vi "Loop Async.vi"(10 "ExecAnchor":refnum<class "ExecAnchor.lvclass">, 11 "HistorianCharting in":refnum<class "HistorianCharting.lvclass">) -> ()   [LabVIEW 2020, in "VolatusGUIElements.lvlib" / "HistorianCharting.lvclass"]
uses:
  HistorianCharting.lvclass
  lv-exec-anchor/ExecAnchor/ExecAnchor.lvclass
  HistorianCharting.lvclass/HistorianCharting.ctl
  <vilib>/dlg_ctls.llb/Space Constant.vi
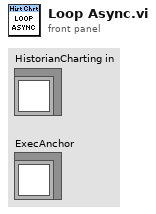
[diagram p1: front panel]
types:
  T1 = cluster{"Event Reg":refnum<event-registration>, "Event Reg":refnum<event-registration>, "Group Events":refnum<event-registration>}
  T2 = typedef "VolatusGUIElements.lvlib/HistorianCharting.lvclass/Buffer Info.ctl" = cluster{"Buffer":refnum<class "Group Buffer DBL.lvclass">, "Channels":string[], "Plot Indices":i32[]}
  T3 = typedef "VolatusGUI.lvlib/Historian Charting Manager.lvclass/Plot Group Config.ctl" = cluster{"Name":string, "X-Axis Type":T4, "X-Axis Channel":string, "Plots":T5[], "Lock Now":bool, "Time":string, "Swap Axes":bool}
  T4 = typedef "VolatusGUI.lvlib/Historian Charting Manager.lvclass/X-Axis Type.ctl" = enum16{"Time", "Channel"}
  T5 = typedef "VolatusGUI.lvlib/Historian Charting Manager.lvclass/Plot Config.ctl" = cluster{"Channel":string, "Visible":bool, "Color":u32, "Scale":T6}
  T6 = typedef "VolatusGUI.lvlib/Historian Charting Manager.lvclass/Scale.ctl" = enum16{"Left", "Right"}
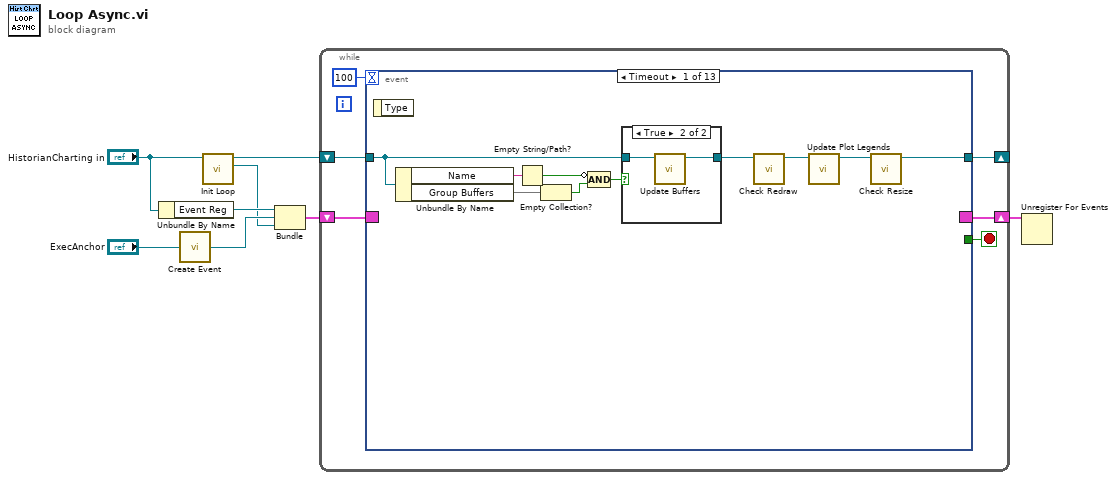
[diagram p0: block diagram]
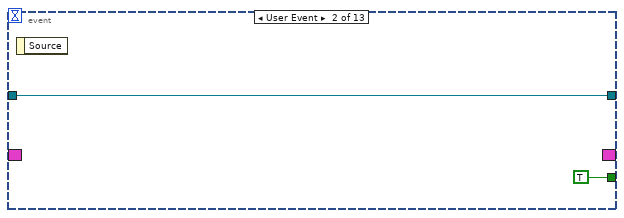
[diagram p3: hidden frame]
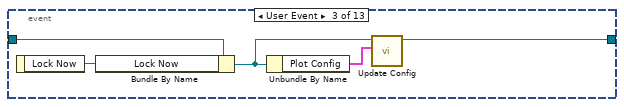
[diagram p4: hidden frame]
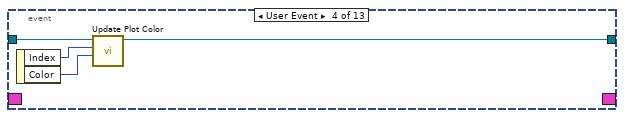
[diagram p5: hidden frame]
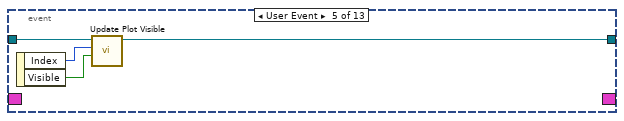
[diagram p6: hidden frame]
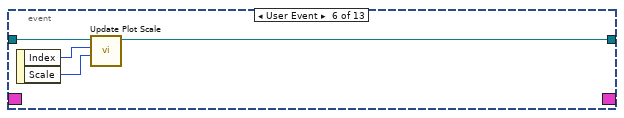
[diagram p7: hidden frame]
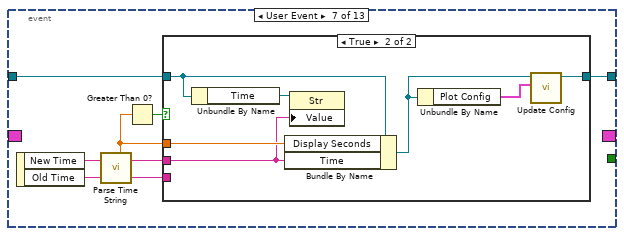
[diagram p8: hidden frame]
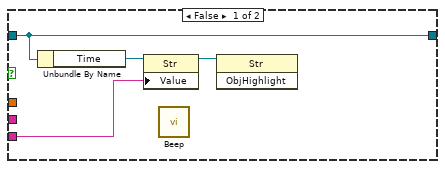
[diagram p9: hidden frame]
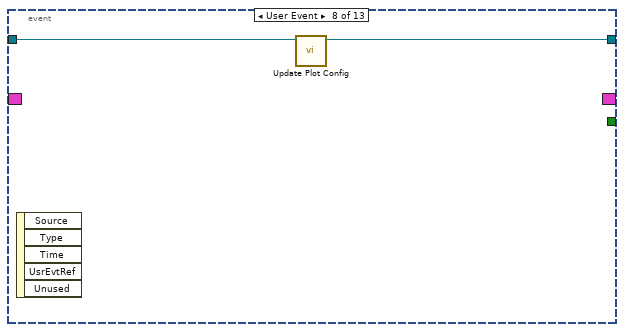
[diagram p10: hidden frame]
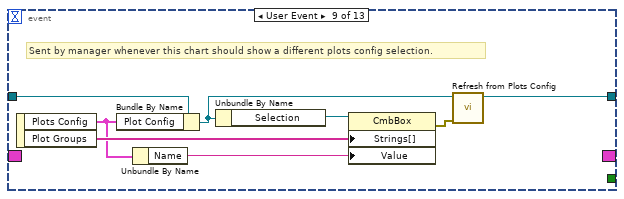
[diagram p11: hidden frame]
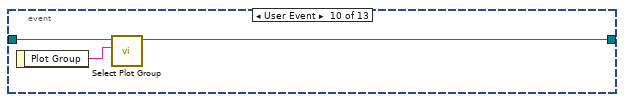
[diagram p12: hidden frame]
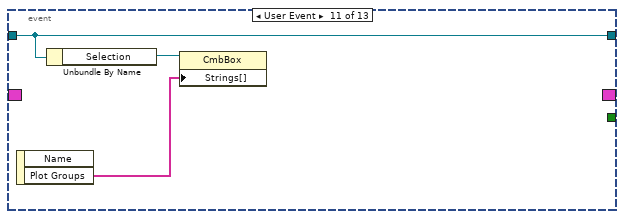
[diagram p13: hidden frame]
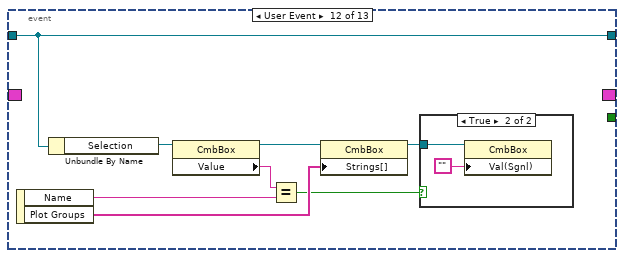
[diagram p14: hidden frame]
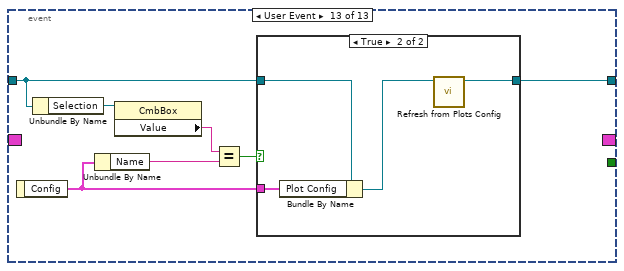
[diagram p16: hidden frame]
diagram:
  n1 = Unbundle By Name("HistorianCharting in") -> ("Event Reg"=w6:refnum<event-registration>)
  n2 = call "Create Event.vi"("ExecAnchor in"="ExecAnchor") -> ("Event Reg"=w5:refnum<event-registration>)  [unwired: 3 in, 1 out]
  n3 = call "Init Loop.vi"("HistorianCharting in"="HistorianCharting in") -> ("Group Events"=w1:refnum<event-registration>, "HistorianCharting out"=w2:refnum<class "HistorianCharting.lvclass">)  [unwired: 8 in, 1 out]
  n4 = Bundle("Event Reg"=w6, "Event Reg"=w5, "Group Events"=w1) -> (w4:T1)  [unwired: 1 in]
  n5 = while {
    shift-right: [w12] -> _
    shift-left: w2 -> [w13]
    shift-right: [w10] -> w3
    shift-left: w4 -> [w11]
    stop <- w9 stop-if-true
    n6 = event shown="[0] Timeout" {
      selector: w11 -> [_ _ _ _ _ _ _ _ _ _ _ _ _]
      dyn-events: [_ _ _ _ _ _ _ _ _ _ _ _ _] -> w10
      timeout: 100 -> [_ _ _ _ _ _ _ _ _ _ _ _ _]
      tunnel: w13 -> [w18 w29 w34 w38 w42 w46 w49 w66 w74 w77 w80 w87 w94]
      tunnel: [w15 w29 w31 w37 w41 w45 w48 w65 w73 w75 w80 w87 w91] -> w12
      tunnel: [_ TRUE _ _ _ _ _ _ _ _ _ _ _] -> w9
      event Timeout {
        n7 = event-data() -> ()  [unwired: 1 in, 1 out]
        n8 = Unbundle By Name(w18) -> ("Name"=w22:string, "Group Buffers"=w21:map{string, T2})
        n9 = Empty String/Path?(string/path=w22) -> (empty?=w20:bool)
        n10 = Empty Collection?(1:w21) -> (0:w19:bool)
        n11 = Compound Arithmetic op=AND(invert w20, w19) -> (w17:bool)
        n12 = case shown="True" w17 {
          tunnel: w18 -> [w25 w27]
          tunnel: [w25 w26] -> w16
          frame False {
          }
          frame True {
            n13 = call "Update Buffers.vi"("HistorianCharting in"=w27) -> ("HistorianCharting out"=w26:refnum<class "HistorianCharting.lvclass">)  [unwired: 9 in, 1 out]
          }
        }
        n14 = call "Check Redraw.vi"("HistorianCharting in"=w16) -> ("HistorianCharting out"=w24:refnum<class "HistorianCharting.lvclass">)  [unwired: 9 in, 1 out]
        n15 = call "Update Plot Legends.vi"("HistorianCharting in"=w24) -> ("HistorianCharting out"=w23:refnum<class "HistorianCharting.lvclass">)  [unwired: 9 in, 1 out]
        n16 = call "Check Resize.vi"("HistorianCharting in"=w23) -> ("HistorianCharting out"=w15:refnum<class "HistorianCharting.lvclass">)  [unwired: 9 in, 1 out]
      }
      event User Event {
        n17 = event-data() -> ()  [unwired: 1 in, 1 out]
      }
      event User Event {
        n18 = event-data() -> ("Lock Now"=w33:bool)  [unwired: 1 in]
        n19 = Bundle By Name(cluster=w34, "Lock Now"=w33) -> (w32:refnum<class "HistorianCharting.lvclass">)
        n20 = Unbundle By Name(w32) -> ("Plot Config"=w30:T3)
        n21 = call "Update Config.vi"("Config"=w30, "HistorianCharting in"=w32) -> ("HistorianCharting out"=w31:refnum<class "HistorianCharting.lvclass">)  [unwired: 8 in, 1 out]
      }
      event User Event {
        n22 = event-data() -> ("Index"=w36:i32, "Color"=w35:u32)  [unwired: 1 in]
        n23 = call "Update Plot Color.vi"("Color"=w35, "Index"=w36, "HistorianCharting in"=w38) -> ("HistorianCharting out"=w37:refnum<class "HistorianCharting.lvclass">)  [unwired: 7 in, 1 out]
      }
      event User Event {
        n24 = event-data() -> ("Index"=w40:i32, "Visible"=w39:bool)  [unwired: 1 in]
        n25 = call "Update Plot Visible.vi"("Visible"=w39, "Index"=w40, "HistorianCharting in"=w42) -> ("HistorianCharting out"=w41:refnum<class "HistorianCharting.lvclass">)  [unwired: 7 in, 1 out]
      }
      event User Event {
        n26 = event-data() -> ("Index"=w44:i32, "Scale"=w43:T6)  [unwired: 1 in]
        n27 = call "Update Plot Scale.vi"("Scale"=w43, "Index"=w44, "HistorianCharting in"=w46) -> ("HistorianCharting out"=w45:refnum<class "HistorianCharting.lvclass">)  [unwired: 7 in, 1 out]
      }
      event User Event {
        n28 = event-data() -> ("New Time"=w53:string, "Old Time"=w47:string)  [unwired: 1 in]
        n29 = call "Parse Time String.vi"("Time String"=w53) -> ("Seconds"=w51:dbl, "Normalized String"=w52:string)  [unwired: 5 in]
        n30 = Greater Than 0?(x=w51) -> (x > 0?=w50:bool)
        n31 = case shown="True" w50 {
          tunnel: w52 -> [_ w61]
          tunnel: w51 -> [_ w64]
          tunnel: w49 -> [w57 w62]
          tunnel: [w57 w60] -> w48
          tunnel: w47 -> [w54 _]
          frame False {
            n32 = Unbundle By Name(w57) -> ("Time"=w56:refnum<vi>)
            n33 = property class="Str"(reference=w56, "Value"=w54) -> (reference out=w55:refnum<vi>)  [unwired: 1 in, 1 out]
            n34 = call <vilib>:"Beep.vi"() -> ()  [unwired: 12 in]
            n35 = invoke class="Str" method="ObjHighlight"(reference=w55) -> ()  [unwired: 2 in, 3 out]
          }
          frame True {
            n36 = Unbundle By Name(w62) -> ("Time"=w63:refnum<vi>)
            n37 = Bundle By Name(cluster=w62, "Display Seconds"=w64, "Time"=w61) -> (w59:refnum<class "HistorianCharting.lvclass">)
            n38 = property class="Str"(reference=w63, "Value"=w61) -> ()  [unwired: 1 in, 2 out]
            n39 = Unbundle By Name(w59) -> ("Plot Config"=w58:T3)
            n40 = call "Update Config.vi"("Config"=w58, "HistorianCharting in"=w59) -> ("HistorianCharting out"=w60:refnum<class "HistorianCharting.lvclass">)  [unwired: 8 in, 1 out]
          }
        }
      }
      event User Event {
        n41 = event-data() -> ()  [unwired: 1 in, 5 out]
        n42 = call "Update Plot Config.vi"("HistorianCharting in"=w66) -> ("HistorianCharting out"=w65:refnum<class "HistorianCharting.lvclass">)  [unwired: 9 in, 1 out]
      }
      event User Event {
        # "Sent by manager whenever this chart should show a different plots config selection."
        n43 = event-data() -> ("Plots Config"=w68:T3, "Plot Groups"=w69:string[])  [unwired: 1 in]
        n44 = Bundle By Name(cluster=w74, "Plot Config"=w68) -> (w70:refnum<class "HistorianCharting.lvclass">)
        n45 = Unbundle By Name(w68) -> ("Name"=w67:string)
        n46 = Unbundle By Name(w70) -> ("Selection"=w72:refnum<vi>)
        n47 = property class="CmbBox"(reference=w72, "Strings[]"=w69, "Value"=w67) -> (error out=w71:errorcluster)  [unwired: 1 in, 1 out]
        n48 = call "Refresh from Plots Config.vi"("error in (no error)"=w71, "HistorianCharting in"=w70) -> ("HistorianCharting out"=w73:refnum<class "HistorianCharting.lvclass">)  [unwired: 8 in, 1 out]
      }
      event User Event {
        n49 = event-data() -> ("Plot Group"=w76:string)  [unwired: 1 in]
        n50 = call "Select Plot Group.vi"("Plot Group"=w76, "HistorianCharting in"=w77) -> ("HistorianCharting out"=w75:refnum<class "HistorianCharting.lvclass">)  [unwired: 8 in, 1 out]
      }
      event User Event {
        n51 = event-data() -> ("Plot Groups"=w78:string[])  [unwired: 1 in, 1 out]
        n52 = Unbundle By Name(w80) -> ("Selection"=w79:refnum<vi>)
        n53 = property class="CmbBox"(reference=w79, "Strings[]"=w78) -> ()  [unwired: 1 in, 2 out]
      }
      event User Event {
        n54 = event-data() -> ("Name"=w84:string, "Plot Groups"=w83:string[])  [unwired: 1 in]
        n55 = Unbundle By Name(w87) -> ("Selection"=w88:refnum<vi>)
        n56 = property class="CmbBox"(reference=w88) -> (reference out=w86:refnum<vi>, "Value"=w85:string)  [unwired: 1 in, 1 out]
        n57 = Equal?(x=w85, y=w84) -> (x = y?=w81:bool)
        n58 = property class="CmbBox"(reference=w86, "Strings[]"=w83) -> (reference out=w82:refnum<vi>)  [unwired: 1 in, 1 out]
        n59 = case shown="True" w81 {
          tunnel: w82 -> [_ w90]
          frame False {
          }
          frame True {
            n60 = property class="CmbBox"(reference=w90, "Val(Sgnl)"="") -> ()  [unwired: 1 in, 2 out]
          }
        }
      }
      event User Event {
        n61 = event-data() -> ("Config"=w92:T3)  [unwired: 1 in]
        n62 = Unbundle By Name(w94) -> ("Selection"=w97:refnum<vi>)
        n63 = Unbundle By Name(w92) -> ("Name"=w95:string)
        n64 = property class="CmbBox"(reference=w97) -> ("Value"=w96:string)  [unwired: 1 in, 2 out]
        n65 = Equal?(x=w96, y=w95) -> (x = y?=w93:bool)
        n66 = case shown="True" w93 {
          tunnel: w94 -> [w98 w102]
          tunnel: w92 -> [_ w101]
          tunnel: [w98 w99] -> w91
          frame False {
          }
          frame True {
            n67 = Bundle By Name(cluster=w102, "Plot Config"=w101) -> (w100:refnum<class "HistorianCharting.lvclass">)
            n68 = call "Refresh from Plots Config.vi"("HistorianCharting in"=w100) -> ("HistorianCharting out"=w99:refnum<class "HistorianCharting.lvclass">)  [unwired: 9 in, 1 out]
          }
        }
      }
    }
  }
  n69 = Unregister For Events(event registration refnum=w3) -> ()  [unwired: 1 in, 1 out]
